vi "append to temp log file.vi"(0 "T cont":T1 {"utility"."therm volt" format="%_6g"; "utility"."heat volt in" format="%_6g"; "utility"."heat volt out" format="%_6g"; "utility"."power out" format="%_6g"; "utility"."H Vmax" format="%_6g"; "exec"."man power" format="%_6g"; "exec"."exec setpoint" format="%_6g"; "T params"."Settle Time" step=1.0; "T params"."Settle Bandwidth" step=0.01; "T params"."Derivative Tme" step=0.01; "T params"."Integral Time" step=1.0; "T params"."Control Bandwidth" step=0.1; "T params"."Setpoint" step=0.1; "T status"."Setpoint" format="%_6g"; "T status"."Power" format="%_6g"; "T status"."Temp" format="%_6g"}, 7 "# to add":i32=100, 11 "error in (no error)":errorcluster, 12 "T log file exists":bool, 13 "temp log file path":path) -> (15 "error out":errorcluster)   [LabVIEW 2019]
doc: "This subVI appends data to the temperature parameters log of the bug experiment.\n\nIt waits for the data log to reach \"# to add\" and then adds the data to the file, and clears then clears array.\n\nThe DAQ state machine will continue to populate the array a row at a time until the limit is reached again, and more data is added to the file.\n\nPaul K Dixon\nP3600\nCSUSB Physics"
uses:
  typedefs/temp cont cluster.ctl
  typedefs/temp exec cluster.ctl
  typedefs/temp mode enum.ctl
  typedefs/temp indicator.ctl
  typedefs/temp control status.ctl
  typedefs/PID control parameters.ctl
  typedefs/temp cont utility.ctl
  <vilib>/Utility/file.llb/Write Delimited Spreadsheet (DBL).vi
  globals/Bug temp globals.vi
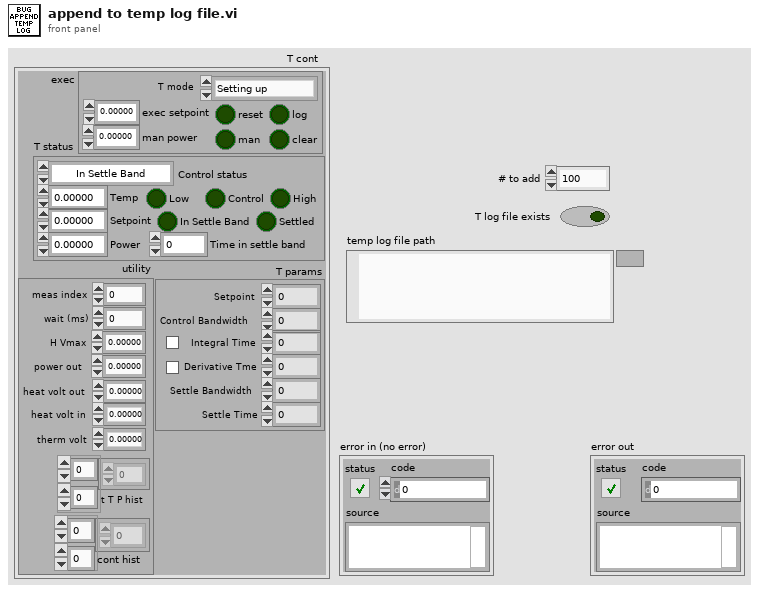
[diagram p1: front panel]
types:
  T1 = typedef "temp cont cluster.ctl" = cluster{"exec":T2, "T status":T4, "T params":T6, "utility":T7}
  T2 = typedef "temp exec cluster.ctl" = cluster{"T mode":T3, "exec setpoint":dbl, "reset":bool, "man power":dbl, "man":bool, "log":bool, "clear":bool}
  T3 = typedef "temp mode enum.ctl" = enum16{"Setting up", "Listening to exec", "Exit"}
  T4 = typedef "temp indicator.ctl" = cluster{"Control status":T5, "Temp":dbl, "Power":dbl, "Time in settle band":dbl, "Settled":bool, "Low":bool, "High":bool, "Setpoint":dbl, "Control":bool, "In Settle Band":bool}
  T5 = typedef "temp control status.ctl" = enum16{"In Settle Band", "In Control Band", "Below Control Band", "Above Control Band"}
  T6 = typedef "PID control parameters.ctl" = cluster{"Setpoint":dbl, "Control Bandwidth":dbl, "Integral Time":dbl, "Int\nON":bool, "Derivative Tme":dbl, "Der\nON":bool, "Settle Bandwidth":dbl, "Settle Time":dbl}
  T7 = typedef "temp cont utility.ctl" = cluster{"meas index":i32, "wait (ms)":i32, "H Vmax":dbl, "power out":dbl, "heat volt out":dbl, "heat volt in":dbl, "therm volt":dbl, "t T P hist":dbl[][], "cont hist":dbl[][]}
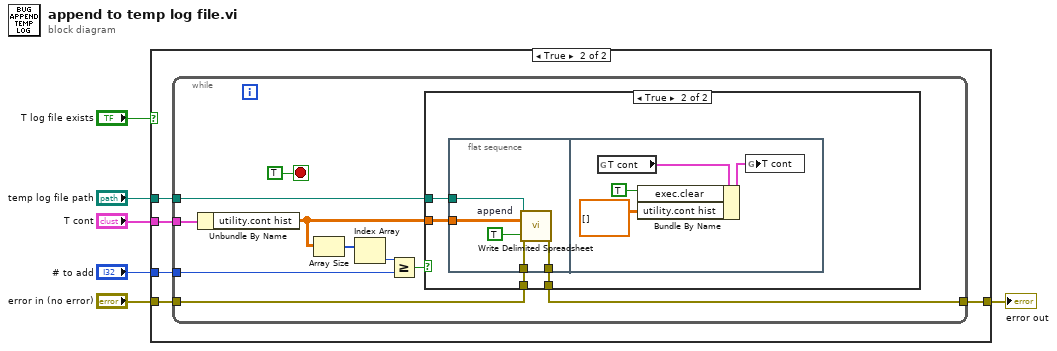
[diagram p0: block diagram]
diagram:
  n1 = case shown="True" "T log file exists" {
    tunnel: "T cont" -> [_ w12]
    tunnel: "# to add" -> [_ w11]
    tunnel: "temp log file path" -> [_ w10]
    tunnel: "error in (no error)" -> [w7 w9]
    tunnel: [w7 w8] -> w3
    frame False {
    }
    frame True {
      n2 = while {
        tunnel: w12 -> [w13]
        tunnel: w11 -> [w19]
        tunnel: w10 -> [w14]
        tunnel: w9 -> [w15]
        tunnel: [w16] -> w8
        stop <- TRUE stop-if-true
        n3 = Unbundle By Name(w13) -> ("utility.cont hist"=w17:dbl[][])
        n4 = Array Size(array=w17) -> (size(s)=w21:i32[])
        n5 = Index Array(array=w21) -> (element=w20:i32)  [unwired: 1 in]
        n6 = Greater Or Equal?(x=w20, y=w19) -> (x >= y?=w18:bool)
        n7 = case shown="True" w18 {
          tunnel: w17 -> [_ w27]
          tunnel: w15 -> [w23 w26]
          tunnel: [w23 w25] -> w16
          tunnel: w14 -> [_ w24]
          frame False {
          }
          frame True {
            n8 = flat-sequence {
              tunnel: w27 -> [w31]
              tunnel: w26 -> [w30]
              tunnel: [w29] -> w25
              tunnel: w24 -> [w28]
              frame #0 {
                w32 = TRUE  # append
                n9 = call-poly <vilib>:"Write Delimited Spreadsheet.vi"("file path (dialog if empty)"=w28, "2D data"=w31, "append to file? (new file:F)"=w32, "error in (no error)"=w30) -> ("error out"=w29:errorcluster)  [unwired: 10 in, 1 out]
              }
              frame #1 {
                n10 = global read "Bug temp globals.vi" "T cont"() -> (w35:T1)
                n11 = Bundle By Name(cluster=w35, "exec.clear"=TRUE, "utility.cont hist"=dbl[][] [] ("temp cont hist")) -> (w36:T1)
                n12 = global write "Bug temp globals.vi" "T cont"(w36) -> ()
              }
            }
          }
        }
      }
    }
  }
  "error out" <- w3
